vi "Send.vi"(7 "Authorization in":refnum<class "Authorization.lvclass">, 8 "error in (no error)":errorcluster, 10 "Google":refnum<class "Google.lvclass">, 11 "Gmail in":refnum<class "Gmail.lvclass">) -> (0 "error out":errorcluster, 3 "Gmail out":refnum<class "Gmail.lvclass">, 5 "Authorization":refnum<class "Authorization.lvclass">)   [LabVIEW 2020, in "Gmail API.lvlib" / "Gmail.lvclass"]
doc: "Sends the email using the provided authorization. An initialized Google OAuth2 instance must be provided to automatically refresh the authorization if it has expired. A refresh does not require user interaction but if the refresh fails the send will not be attempted and an error will be returned."
uses:
  Gmail.lvclass
  <vilib>/IlluminatedG/IG OAuth2/OAuth2/Authorization/Authorization.lvclass
  <vilib>/IlluminatedG/IG OAuth2/OAuth2/Google/Google.lvclass
  <vilib>/IlluminatedG/lv-web-crypto/lv-base64/Variant.ctl
  <vilib>/httpClient/POSTBuffer.vi
  <vilib>/IlluminatedG/lv-web-crypto/lv-base64/Base64.lvlib
  <vilib>/httpClient/LabVIEWHTTPClient.lvlib
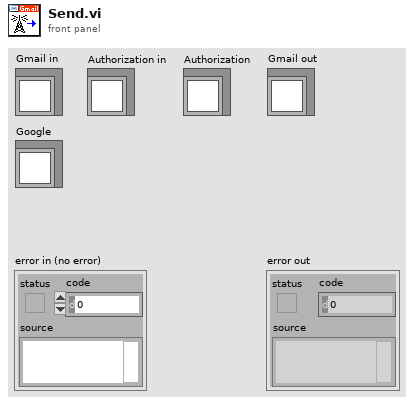
[diagram p1: front panel]
types:
  T1 = typedef "Base64.lvlib/Variant.ctl" = enum16{"Base64", "Base64-URL"}
  T2 = typedef "LabVIEWHTTPClient.lvlib/ClientHandle.ctl" = refnum<k1>
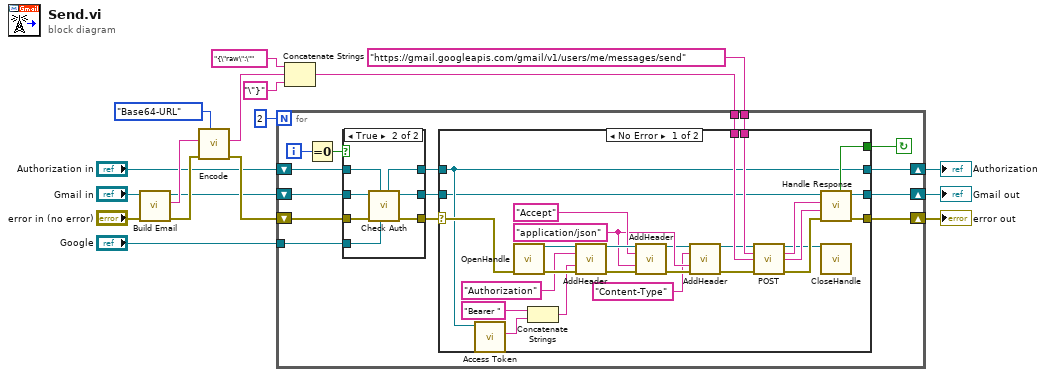
[diagram p0: block diagram]
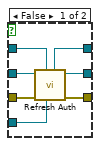
[diagram p3: hidden frame]
diagram:
  n1 = call "Build Email.vi"("error in (no error)"="error in (no error)", "Gmail in"="Gmail in") -> ("error out"=w14:errorcluster, "Email"=w16:string, "Gmail out"=w6:refnum<class "Gmail.lvclass">)  [unwired: 7 in]
  n2 = call <vilib>:"Encode.vi"("Variant (Base64)"=Variant."Base64-URL", "error in (no error)"=w14, "string in (not encoded)"=w16) -> ("error out"=w8:errorcluster, "string out (base64-encoded)"=w12:string)  [unwired: 7 in]
  n3 = Concatenate Strings("{\"raw\":\"", w12, "\"}" ("string")) -> (w9:string)
  n4 = for {
    N: 2 -> [_]
    tunnel: "https://gmail.googleapis.com/gmail/v1/users/me/messages/send" ("url") -> [w33]
    tunnel: w9 -> [w32]
    shift-right: [w25] -> w5
    shift-left: w6 -> [w29]
    shift-right: [w24] -> w4
    shift-left: w8 -> [w28]
    shift-right: [w20] -> w2
    shift-left: "Authorization in" -> [w22]
    tunnel: "Google" -> [w19]
    i -> [w31]
    stop <- w23 continue-if-true
    n5 = Equal To 0?(x=w31) -> (x = 0?=w30:bool)
    n6 = case shown="True" w30 {
      tunnel: w29 -> [w70 w77]
      tunnel: w28 -> [w69 w76]
      tunnel: [w68 w75] -> w27
      tunnel: [w67 w74] -> w26
      tunnel: w22 -> [w66 w73]
      tunnel: [w65 w72] -> w21
      tunnel: w19 -> [w64 w71]
      frame False {
        n7 = call "Refresh Auth.vi"("Google"=w64, "Authorization in"=w66, "error in (no error)"=w69, "Gmail in"=w70) -> ("error out"=w68:errorcluster, "Gmail out"=w67:refnum<class "Gmail.lvclass">, "Authorization"=w65:refnum<class "Authorization.lvclass">)  [unwired: 5 in]
      }
      frame True {
        n8 = call "Check Auth.vi"("Google"=w71, "Authorization in"=w73, "error in (no error)"=w76, "Gmail in"=w77) -> ("error out"=w75:errorcluster, "Gmail out"=w74:refnum<class "Gmail.lvclass">, "Authorization"=w72:refnum<class "Authorization.lvclass">)  [unwired: 5 in]
      }
    }
    n9 = case shown="No Error" w27 {
      selector: w27 -> [w59 w62]
      tunnel: w33 -> [w58 _]
      tunnel: w32 -> [w57 _]
      tunnel: w26 -> [w34 w63]
      tunnel: [w42 w63] -> w25
      tunnel: [w41 w62] -> w24
      tunnel: [w38 _] -> w23
      tunnel: w21 -> [w36 w61]
      tunnel: [w36 w61] -> w20
      frame No Error {
        w48 = "application/json"
        n10 = call <vilib>:"Access Token.vi"("Authorization in"=w36) -> ("Access Token"=w37:string)  [unwired: 10 in]
        n11 = call <vilib>:"OpenHandle.vi"("error in (no error)"=w59) -> ("client handle out"=w56:T2, "error out"=w55:errorcluster)  [unwired: 13 in]
        n12 = Concatenate Strings("Bearer ", w37) -> (w52:string)
        n13 = call <vilib>:"AddHeader.vi"("client handle"=w56, "header"="Authorization", "value"=w52, "error in (no error)"=w55) -> ("client handle out"=w51:T2, "error out"=w50:errorcluster)  [unwired: 10 in]
        n14 = call <vilib>:"AddHeader.vi"("client handle"=w51, "header"="Accept", "value"=w48, "error in (no error)"=w50) -> ("client handle out"=w47:T2, "error out"=w46:errorcluster)  [unwired: 10 in]
        n15 = call <vilib>:"AddHeader.vi"("client handle"=w47, "header"="Content-Type", "value"=w48, "error in (no error)"=w46) -> ("client handle out"=w44:T2, "error out"=w43:errorcluster)  [unwired: 10 in]
        n16 = call-poly <vilib>:"POST.vi"("client handle"=w44, "url"=w58, "buffer"=w57, "error in (no error)"=w43) -> ("client handle out"=w35:T2, "headers"=w40:string, "body"=w39:string, "error out"=w60:errorcluster)  [unwired: 8 in]
        n17 = call "Handle Response.vi"("error in (no error)"=w60, "Body"=w39, "Headers"=w40, "Gmail in"=w34) -> ("error out"=w41:errorcluster, "Gmail out"=w42:refnum<class "Gmail.lvclass">, "Refresh?"=w38:bool)  [unwired: 5 in]
        n18 = call <vilib>:"CloseHandle.vi"("client handle"=w35) -> ()  [unwired: 14 in, 1 out]
      }
      frame Error {
      }
    }
  }
  "error out" <- w4
  "Gmail out" <- w5
  "Authorization" <- w2
